vi "Display results.vi"(0 "Array":cluster{i32, dbl}[](array[cluster]), 1 "Array 3":dbl[](array[numeric]), 2 "Array 2":i32[](array[numeric])) -> ()   [LabVIEW 2009]
uses:
  <vilib>/Utility/file.llb/Write To Spreadsheet File (DBL).vi
panel:
  in  "Save data?":bool
  in  "stop":bool
  out "XY Graph":cluster{i32, dbl}[](graph)
  out "N_spots     Time":dbl[][](array[numeric])
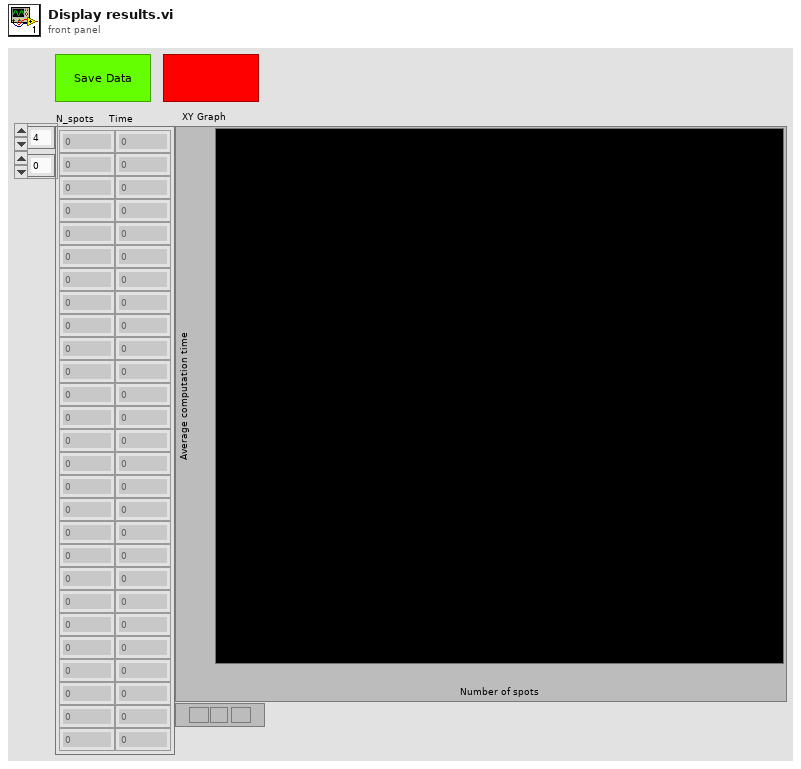
[diagram p1: front panel]
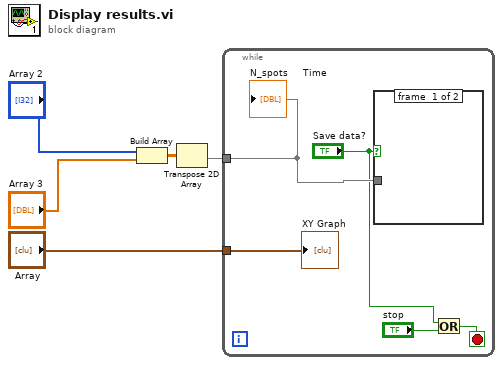
[diagram p0: block diagram]
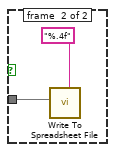
[diagram p2: hidden frame]
diagram:
  n1 = Build Array("Array 2", "Array 3") -> (w4:dbl[][])
  n2 = Transpose 2D Array(2D array=w4) -> (transposed array=w5:dbl[][])
  n3 = while {
    tunnel: "Array" -> [w10]
    tunnel: w5 -> [w9]
    stop <- w7 stop-if-true
    n4 = case shown="True" "Save data?" {
      tunnel: w9 -> [_ w12]
      frame #0 {
      }
      frame #1 {
        n5 = call-poly <vilib>:"Write To Spreadsheet File.vi"("format (%.3f)"="%.4f", "2D data"=w12) -> ()  [unwired: 6 in, 1 out]
      }
    }
    n6 = Or(x="Save data?", y="stop") -> (x .or. y?=w7:bool)
    "N_spots     Time" <- w9
    "XY Graph" <- w10
  }
